vi "PNDT - calc data reduction.vi"(10 "sub-sampling":T1=1 items=["", "1:1", "2:1", "3:1", "4:1", "5:1", "6:1", "7:1", "8:1", "9:1", "10:1"], 11 "data length":i32) -> (2 "sampling length":i32, 3 "no. of points":i32)   [LabVIEW 2026, in "MicroPulse_Driver.lvlib"]
uses:
  MicroPulse_Driver.lvlib
  Public/Data/Datatypes/PNDT - subsampling.ctl
  <instrlib>/Micropulse/Micropulse.lvlib
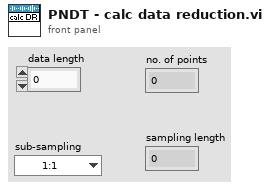
[diagram p1: front panel]
types:
  T1 = typedef "Micropulse.lvlib/PNDT - subsampling.ctl" = u16
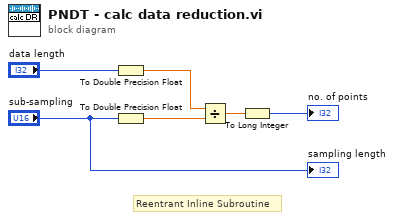
[diagram p0: block diagram]
diagram:
  # "Reentrant Inline Subroutine"
  n1 = To Double Precision Float(number="data length") -> (double precision float=w4:dbl)
  n2 = To Double Precision Float(number="sub-sampling") -> (double precision float=w2:dbl)
  n3 = Divide(x=w4, y=w2) -> (x/y=w5:dbl)
  n4 = To Long Integer(number=w5) -> (32bit integer=→"no. of points":i32)
  "sampling length" <- "sub-sampling"
